vi "SetSingleAttackZone.vi"(8 "error in (no error)":errorcluster, 10 "FieldRef":refnum<class "Field.lvclass">, 11 "object in":refnum<class "Zone.lvclass">) -> (0 "error out":errorcluster, 3 "object out":refnum<class "Zone.lvclass">)   [LabVIEW 2023, in "Zone.lvclass"]
uses:
  Zone.lvclass
  Field_class/Field.lvclass
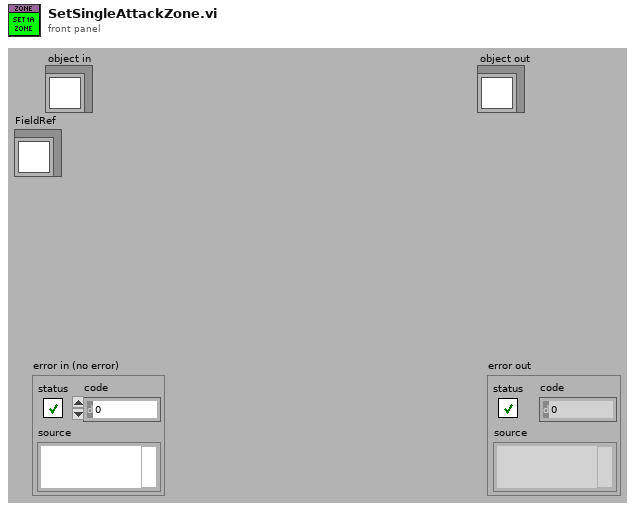
[diagram p1: front panel]
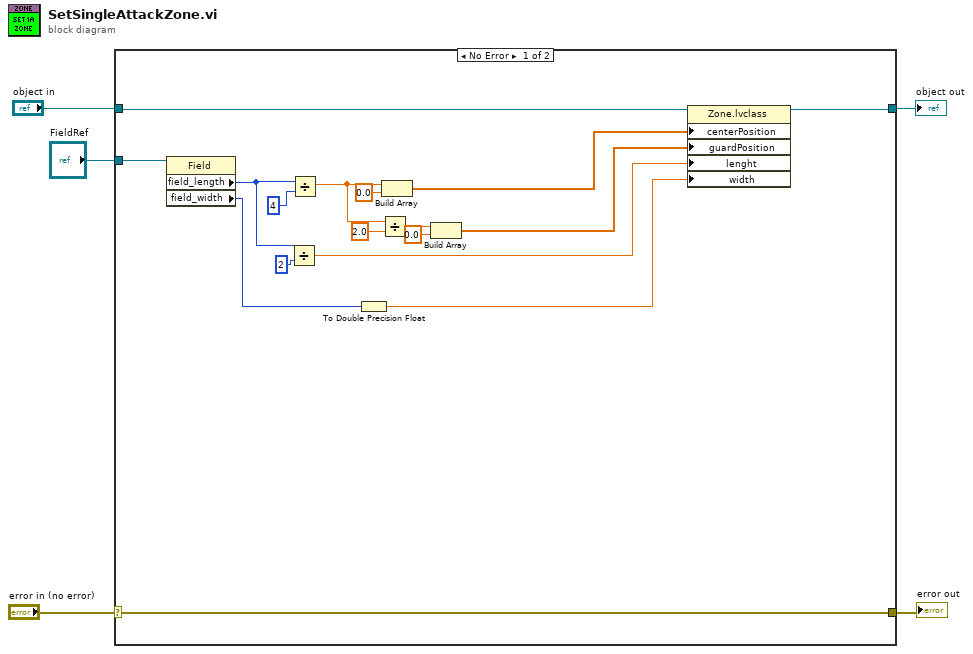
[diagram p0: block diagram]
diagram:
  n1 = case shown="No Error" "error in (no error)" {
    selector: "error in (no error)" -> [w22 w24]
    tunnel: [w22 w24] -> w4
    tunnel: [w21 w23] -> w2
    tunnel: "object in" -> [w20 w23]
    tunnel: "FieldRef" -> [w19 _]
    frame No Error {
      n2 = property class="Field"(reference=w19) -> ("field_length"=w11:i32, "field_width"=w8:i32)  [unwired: 1 in, 2 out]
      n3 = Divide(x=w11, y=2) -> (x/y=w9:dbl)
      n4 = Divide(x=w11, y=4) -> (x/y=w15:dbl)
      n5 = To Double Precision Float(number=w8) -> (double precision float=w7:dbl)
      n6 = Divide(x=w15, y=2.0) -> (x/y=w13:dbl)
      n7 = Build Array(w15, 0.0 ("element")) -> (w16:dbl[])
      n8 = Build Array(w13, 0.0 ("element")) -> (w6:dbl[])
      n9 = property class="Zone.lvclass"(reference=w20, "centerPosition"=w16, "guardPosition"=w6, "lenght"=w9, "width"=w7) -> (reference out=w21:refnum<class "Zone.lvclass">)  [unwired: 1 in, 1 out]
    }
    frame Error {
    }
  }
  "error out" <- w4
  "object out" <- w2
